vi "ChipKit Thermistor Read.vi"() -> ()   [LabVIEW 2011, in "LabVIEW Interface for ChipKit.lvlib"]
doc: "An example that uses an Arduino to read the temperature from a thermistor. The user is able to select the supply voltage, paired resistance, analog input pin and units (C, F, K)."
uses:
  <vilib>/LabVIEW Interface for ChipKit/LabVIEW Interface for ChipKit.lvlib
panel:
  in  "VISA resource name":refnum<visa-resource-name>
  in  "Paired Resistance (Ohms)":dbl=10000.0
  out "Temperature":dbl(slide) scale=0.0..100.0
  in  "Units":enum16{"Celsius", "Fahrenheit", "Kelvin"}(ring)
  in  "Thermistor AI Pin":u8=1
  in  "Stop":bool
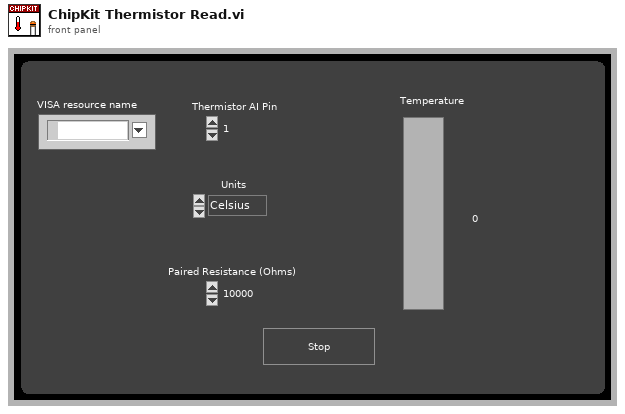
[diagram p1: front panel]
types:
  T1 = typedef "LabVIEW Interface for ChipKit.lvlib/Chipkit Resource.ctl" = cluster{"VISA resource":refnum<visa-resource-name>, "Board Type":T2, "Connection Type":enum8{"USB / Serial"}, "Bytes Per Packet (15)":u8}
  T2 = typedef "LabVIEW Interface for ChipKit.lvlib/Board Type.ctl" = enum16{"Arduino Uno", "Dimuelanove w/Atmega 328", "Mega 2560", "Chipkit Uno32", "Chipkit Max32"}
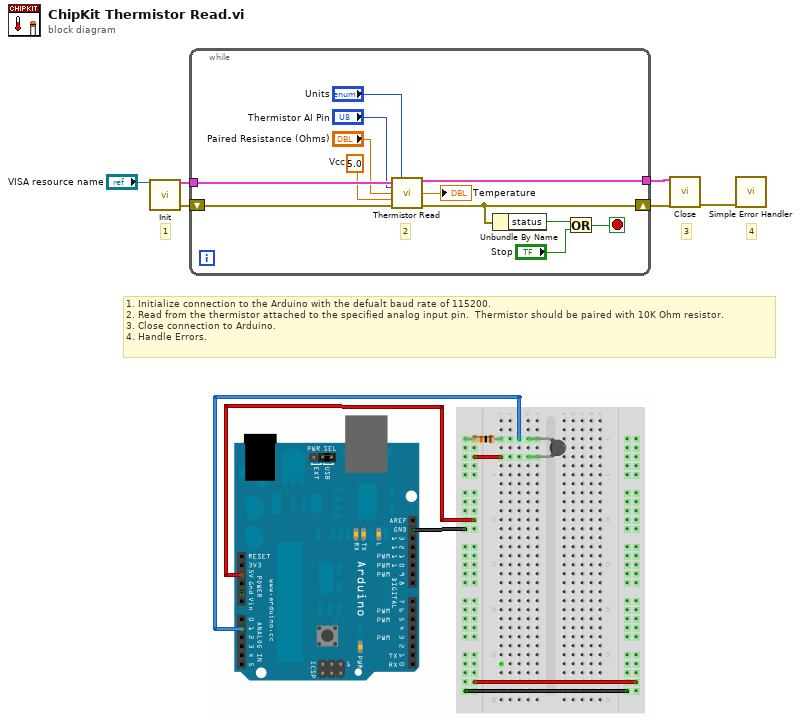
[diagram p0: block diagram]
diagram:
  # "4"
  # "3"
  # "1"
  # "1. Initialize connection to the Arduino with the defualt baud rate of 115200.\n2. Read from the thermistor attached to the specified analog input pin.  Thermistor should be paired with 10K Ohm resistor.\n3. Close connection to Arduino.\n4. Handle Errors."
  n1 = call <vilib>:"Init.vi"("VISA resource"="VISA resource name") -> ("Arduino Resource"=w6:T1, "error out"=w5:errorcluster)  [unwired: 17 in]
  n2 = while {
    tunnel: w6 -> [w16]
    shift-right: [w11] -> w4
    shift-left: w5 -> [w12]
    tunnel: [w9] -> w2
    stop <- w17 stop-if-true
    w13 = 5.0  # Vcc
    # "2"
    n3 = call <vilib>:"Thermistor Read.vi"("Arduino Resource"=w16, "Units (C)"="Units", "Thermistor AI Pin (0)"="Thermistor AI Pin", "Paired Resistance (10K Ohms)"="Paired Resistance (Ohms)", "Vcc (5 v)"=w13, "error in"=w12) -> ("Arduino Resource"=w9:T1, "Temperature"=→"Temperature":dbl, "error out"=w11:errorcluster)  [unwired: 7 in]
    n4 = Unbundle By Name(w11) -> ("status"=w7:bool)
    n5 = Or(x=w7, y="Stop") -> (x .or. y?=w17:bool)
  }
  n6 = call <vilib>:"Close.vi"("Arduino Resource"=w2, "error in"=w4) -> ("error out"=w3:errorcluster)  [unwired: 13 in]
  n7 = call <vilib>:"Simple Error Handler.vi"("error in (no error)"=w3) -> ()  [unwired: 4 in, 5 out]
